vi "PT3_Open.vi"(8 "error in":errorcluster, 11 "File Path":path) -> (0 "error out":errorcluster, 1 "Num Records":i32, 2 "Header":T1, 3 "refnum out":refnum<file>, 4 "Stop After (ms)":i32, 5 "Stop Reason":enum16{"timeover", "manual", "overflow"}(ring))   [LabVIEW 8.6]
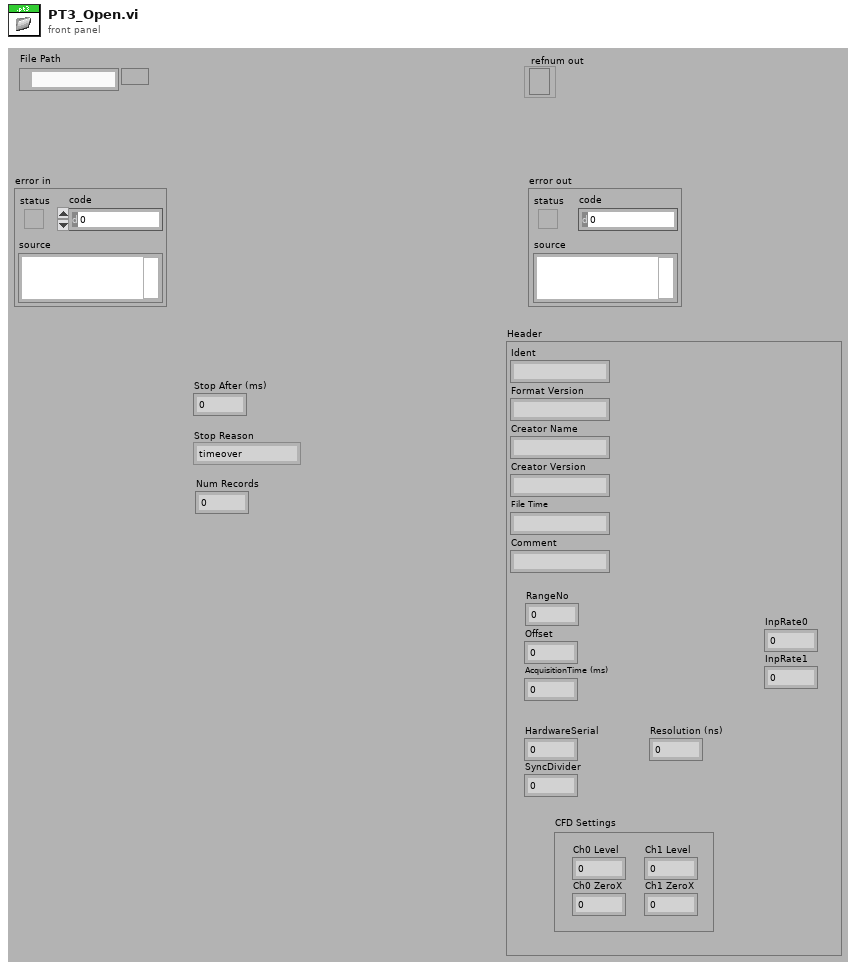
[diagram p1: front panel]
types:
  T1 = cluster{"Ident":string, "Format Version":string, "Creator Name":string, "Creator Version":string, "File Time":string, "Comment":string, "RangeNo":i32, "Offset":i32, "AcquisitionTime (ms)":i32, "HardwareSerial":i32, "SyncDivider":i32, "Resolution (ns)":sgl, "CFD Settings":cluster{"Ch0 Level":i32, "Ch0 ZeroX":i32, "Ch1 Level":i32, "Ch1 ZeroX":i32}, "InpRate0":i32, "InpRate1":i32}
  T2 = enum16{"big-endian, network order", "native, host order", "little-endian"}
  T3 = enum16{"open", "replace", "create", "open or create", "replace or create", "replace or create with confirmation"}
  T4 = cluster{"Strings[0]":string, "Strings[1]":string, "Strings[2]":string, "Strings[3]":string, "Strings[4]":string, "Strings[5]":string}
  T5 = cluster{"[0]":i32, "[1]":i32, "[2]":i32, "[3]":i32, "[4]":i32, "[5]":i32}
  T6 = cluster{"[3]":i32, "[2]":i32, "[5]":i32, "[4]":i32}
  T7 = cluster{"[0]":i32, "[1]":i32, "[2]":i32, "[3]":i32, "[4]":i32, "[5]":i32, "[6]":i32, "[7]":i32, "[8]":i32}
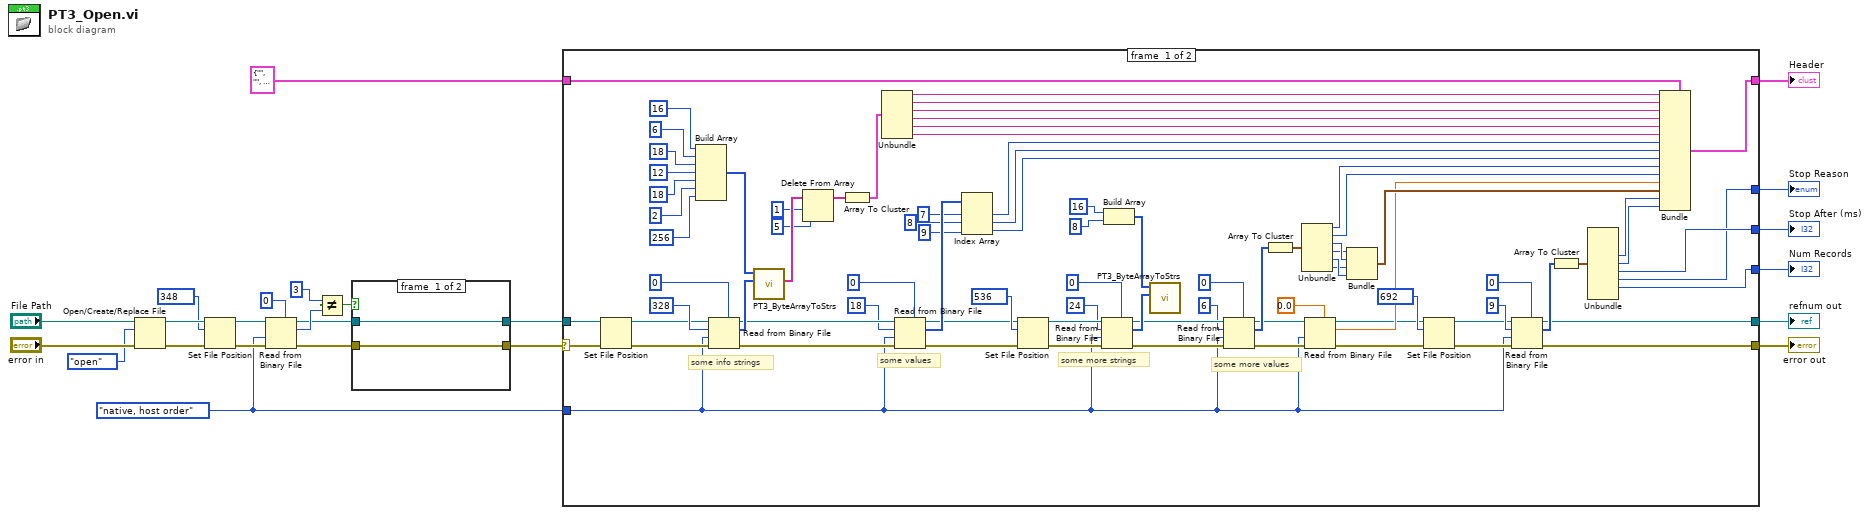
[diagram p0: block diagram]
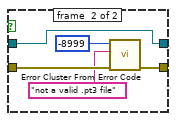
[diagram p2: hidden frame]
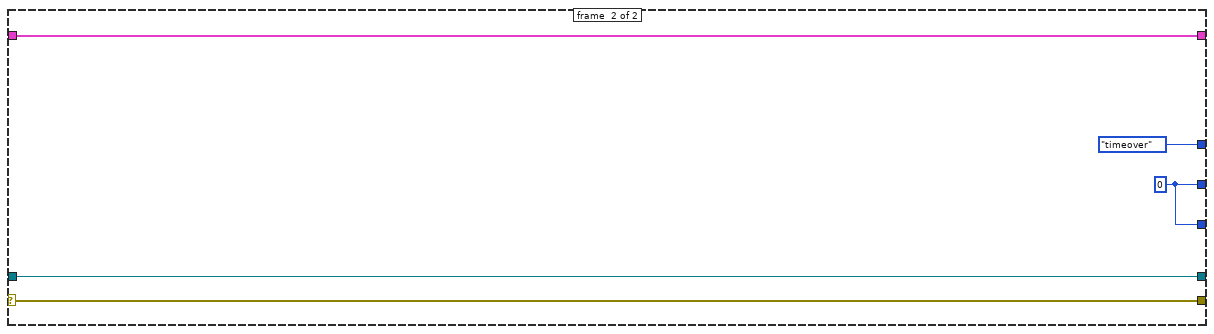
[diagram p3: hidden frame]
diagram:
  w10 = T2."native, host order" ("byte order (0:big-endian, network order)")
  n1 = Open/Create/Replace File(file path (use dialog)="File Path", error in="error in", operation (0:open)=T3."open") -> (refnum out=w13:refnum<file>, error out=w14:errorcluster)  [unwired: 4 out]
  n2 = Set File Position(offset (in bytes) (0)=i64 348, refnum=w13, error in=w14) -> (refnum out=w9:refnum<file>, error out=w11:errorcluster)  [unwired: 1 out]
  n3 = Read from Binary File(5:0, 8:w11, 9:w10, 11:w9) -> (0:w4:errorcluster, 2:w7:i32, 3:w1:refnum<file>)  [unwired: 3 out]
  n4 = Not Equal?(x=3, y=w7) -> (x != y?=w5:bool)
  n5 = case shown="True" w5 {
    tunnel: w4 -> [w26 w31]
    tunnel: [w26 w30] -> w3
    tunnel: [w25 w27] -> w2
    tunnel: w1 -> [w25 w27]
    frame #0 {
    }
    frame #1 {
      n6 = call <vilib>:"Error Cluster From Error Code.vi"("error in (no error)"=w31, "error message (\"\")"="not a valid .pt3 file" ("error message (\"\")"), "error code (0)"=-8999) -> ("error out"=w30:errorcluster)  [unwired: 1 in, 5 out]
    }
  }
  n7 = case shown="No Error" w3 {
    selector: w3 -> [w98 w120]
    tunnel: [w36 w120] -> w21
    tunnel: [w35 w119] -> w20
    tunnel: w2 -> [w96 w119]
    tunnel: w10 -> [w42 _]
    tunnel: [w87 w116] -> w19
    tunnel: [w32 enum16{"timeover", "manual", "overflow"}."timeover" ("Stop Reason")] -> w18
    tunnel: [w34 w117] -> w17
    tunnel: [w33 w117] -> w16
    tunnel: T1 {"Ident"="", "Format Version"="", "Creator Name"="", "Creator Version"="", "File Time"="", "Comment"="", "RangeNo"=0, "Offset"=0, "AcquisitionTime (ms)"=0, "HardwareSerial"=0, "SyncDivider"=0, "Resolution (ns)"=0.0, "CFD Settings"={"Ch0 Level"=0, "Ch0 ZeroX"=0, "Ch1 Level"=0, "Ch1 ZeroX"=0}, "InpRate0"=0, "InpRate1"=0} ("Header") -> [w88 w116]
    frame #0 {
      # "some more values"
      # "some more strings"
      # "some values"
      # "some info strings"
      n8 = Set File Position(refnum=w96, error in=w98) -> (refnum out=w95:refnum<file>, error out=w97:errorcluster)  [unwired: 2 out]
      n9 = Build Array(16 ("Length"), 6 ("Length"), 18 ("Length"), 12 ("Length"), 18 ("Length"), 2 ("Length"), 256 ("Length")) -> (w105:i32[])
      n10 = Read from Binary File(5:u8 0, 8:w97, 9:w42, 10:328 ("count (1)"), 11:w95) -> (0:w100:errorcluster, 2:w113:u8[], 3:w99:refnum<file>)  [unwired: 2 out]
      n11 = call "PT3_ByteArrayToStrs.vi"("Byte Array"=w113, "Lengths"=w105) -> ("Strings"=w104:string[])  [unwired: 9 out]
      n12 = Delete From Array(array=w104, length=1, index=5) -> (array with subset deleted=w101:string[])  [unwired: 1 out]
      n13 = Array To Cluster(array=w101) -> (cluster=w86:T4)
      n14 = Unbundle(w86) -> ("Strings[0]"=w85:string, "Strings[1]"=w84:string, "Strings[2]"=w83:string, "Strings[3]"=w82:string, "Strings[4]"=w81:string, "Strings[5]"=w80:string)
      n15 = Read from Binary File(5:0, 8:w100, 9:w42, 10:18 ("count (1)"), 11:w99) -> (0:w75:errorcluster, 2:w92:i32[], 3:w74:refnum<file>)  [unwired: 2 out]
      n16 = Index Array(array=w92, index #1=7 ("index"), index #2=8 ("index"), index #3=9 ("index")) -> (element #1=w79:i32, element #2=w78:i32, element #3=w77:i32)
      n17 = Set File Position(offset (in bytes) (0)=i64 536, refnum=w74, error in=w75) -> (refnum out=w72:refnum<file>, error out=w73:errorcluster)  [unwired: 1 out]
      n18 = Read from Binary File(5:u8 0, 8:w73, 9:w42, 10:24 ("count (1)"), 11:w72) -> (0:w65:errorcluster, 2:w69:u8[], 3:w64:refnum<file>)  [unwired: 2 out]
      n19 = Build Array(16 ("Length"), 8 ("Length")) -> (w66:i32[])
      n20 = call "PT3_ByteArrayToStrs.vi"("Byte Array"=w69, "Lengths"=w66) -> ()  [unwired: 10 out]
      n21 = Read from Binary File(5:0, 8:w65, 9:w42, 10:6 ("count (1)"), 11:w64) -> (0:w52:errorcluster, 2:w61:i32[], 3:w50:refnum<file>)  [unwired: 2 out]
      n22 = Array To Cluster(array=w61) -> (cluster=w60:T5)
      n23 = Unbundle(w60) -> ("[0]"=w59:i32, "[1]"=w58:i32, "[2]"=w57:i32, "[3]"=w56:i32, "[4]"=w55:i32, "[5]"=w54:i32)
      n24 = Read from Binary File(5:sgl 0.0 ("Resolution (ns)"), 8:w52, 9:w42, 11:w50) -> (0:w47:errorcluster, 2:w49:sgl, 3:w46:refnum<file>)  [unwired: 3 out]
      n25 = Bundle("[3]"=w56, "[2]"=w57, "[5]"=w54, "[4]"=w55) -> (w53:T6)  [unwired: 1 out]
      n26 = Set File Position(offset (in bytes) (0)=i64 692, refnum=w46, error in=w47) -> (refnum out=w41:refnum<file>, error out=w43:errorcluster)  [unwired: 1 out]
      n27 = Read from Binary File(5:0, 8:w43, 9:w42, 10:9 ("count (1)"), 11:w41) -> (0:w36:errorcluster, 2:w39:i32[], 3:w35:refnum<file>)  [unwired: 2 out]
      n28 = Array To Cluster(array=w39) -> (cluster=w40:T7)
      n29 = Unbundle(w40) -> ("[3]"=w38:i32, "[4]"=w37:i32, "[5]"=w34:i32, "[6]"=w32:i32, "[7]"=w33:i32)  [unwired: 4 out]
      n30 = Bundle(cluster=w88, "Ident"=w85, "Format Version"=w84, "Creator Name"=w83, "Creator Version"=w82, "File Time"=w81, "Comment"=w80, "RangeNo"=w79, "Offset"=w78, "AcquisitionTime (ms)"=w77, "HardwareSerial"=w59, "SyncDivider"=w58, "Resolution (ns)"=w49, "CFD Settings"=w53, "InpRate0"=w38, "InpRate1"=w37) -> (w87:T1)
    }
    frame #1 {
      w117 = 0 ("Stop After (ms)")
    }
  }
  "refnum out" <- w20
  "error out" <- w21
  "Header" <- w19
  "Stop Reason" <- w18
  "Stop After (ms)" <- w17
  "Num Records" <- w16
